vi "Edit Options.vi"(6 "Calling VI in":refnum<vi>, 8 "error in (no error)":errorcluster, 11 "Config":T1) -> (0 "error out":errorcluster, 2 "OK?":bool, 3 "Config out":T1)   [LabVIEW 2020, in "VI Properties Editor.lvlib"]
doc: "Displays a window to edit various options present in the tool."
uses:
  VI Properties Editor.lvlib
  CTLs/Config.ctl
  CTLs/Filter Info.ctl
  CTLs/Filter Column.ctl
  CTLs/Filter Type.ctl
panel:
  in  "Tab Control":enum32{"View", "Dialog", "Copyright"}(tab)
  in  "Show Conpane Ctls Only?":bool caption="Show connector pane controls only"
  in  "Format Bold Tags?":bool caption="Format bold text tags"
  in  "Abbreviate Names?":bool caption="Abbreviate names"
  in  "Show Top-Level Ctls Only?":bool caption="Show top-level controls only"
  in  "Confirm Save?":bool caption="Confirm Save action"
  in  "Confirm Save All?":bool caption="Confirm Save All action"
  in  "Confirm Revert?":bool caption="Confirm Revert action"
  in  "Confirm Revert All?":bool caption="Confirm Revert All action"
  in  "Confirm Exit?":bool caption="Confirm Exit with Unsaved Changes action"
  in  "Copyright delimiter":string
  in  "Copyright path":path
  in  "Cancel":bool
  in  "OK":bool
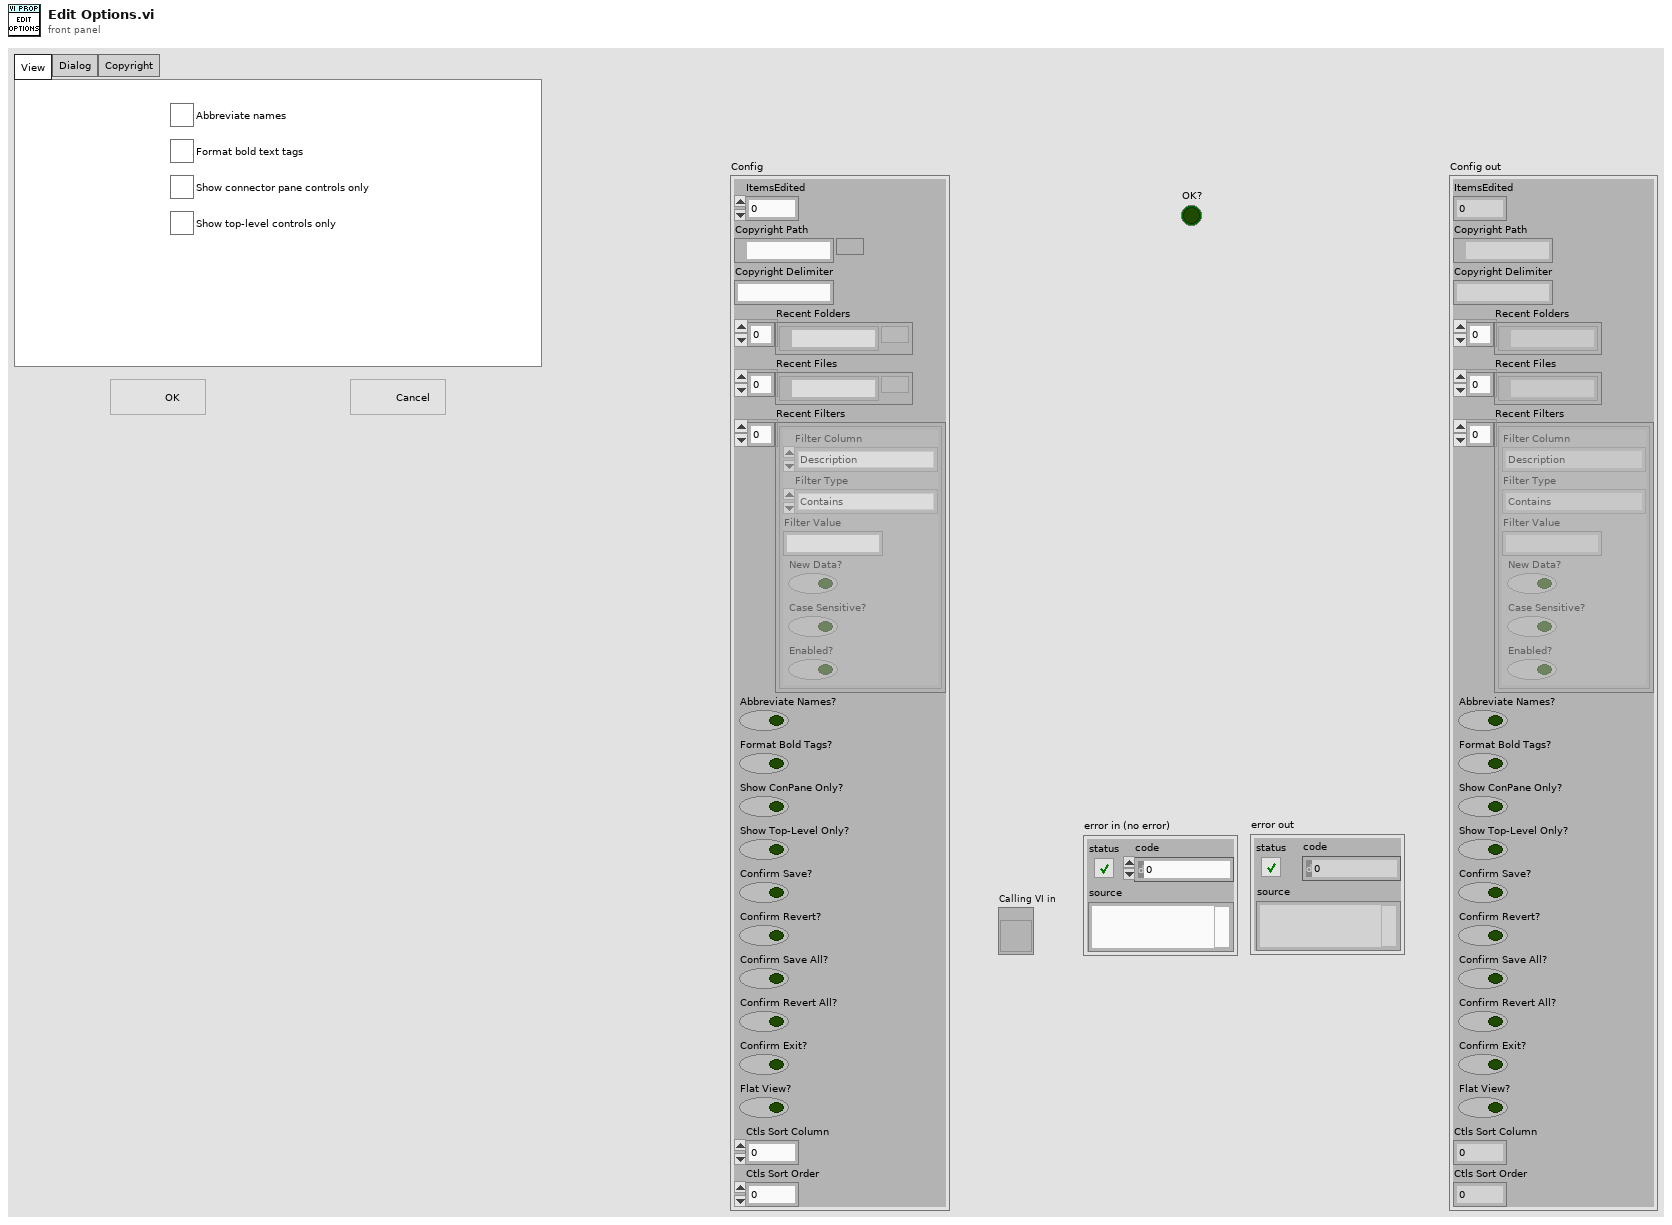
[diagram p1: front panel]
types:
  T1 = typedef "VI Properties Editor.lvlib/Config.ctl" = cluster{"ItemsEdited":u32, "Copyright Path":path, "Copyright Delimiter":string, "Recent Folders":path[], "Recent Files":path[], "Recent Filters":T2[], "Abbreviate Names?":bool, "Format Bold Tags?":bool, "Show ConPane Only?":bool, "Show Top-Level Only?":bool, "Confirm Save?":bool, "Confirm Revert?":bool, "Confirm Save All?":bool, "Confirm Revert All?":bool, "Confirm Exit?":bool, "Flat View?":bool, "Ctls Sort Column":i32, "Ctls Sort Order":i32}
  T2 = typedef "VI Properties Editor.lvlib/Filter Info.ctl" = cluster{"Filter Column":T3, "Filter Type":T4, "Filter Value":string, "New Data?":bool, "Case Sensitive?":bool, "Enabled?":bool}
  T3 = typedef "VI Properties Editor.lvlib/Filter Column.ctl" = enum16{"Name", "Path", "Type", "Window Title", "Description", "Help Path", "Help Tag", "Custom Title?", "Reentrancy", "Inlined?", "Help URL", "Help Type", "Allow Debugging?", "Auto Error Handling?", "Run When Opened?", "Suspend When Called?", "Priority", "Preferred Exec Sytem", "Control Label", "Control Caption", "Control Description", "Control Tip Strip"}
  T4 = typedef "VI Properties Editor.lvlib/Filter Type.ctl" = enum16{"Contains", "Equals", "Starts with", "Ends with", "Is empty", "Does not contain", "Does not equal", "Is not empty"}
  T5 = enum32{"Invalid", "Standard", "Closed", "Hidden", "Minimized", "Maximized"}
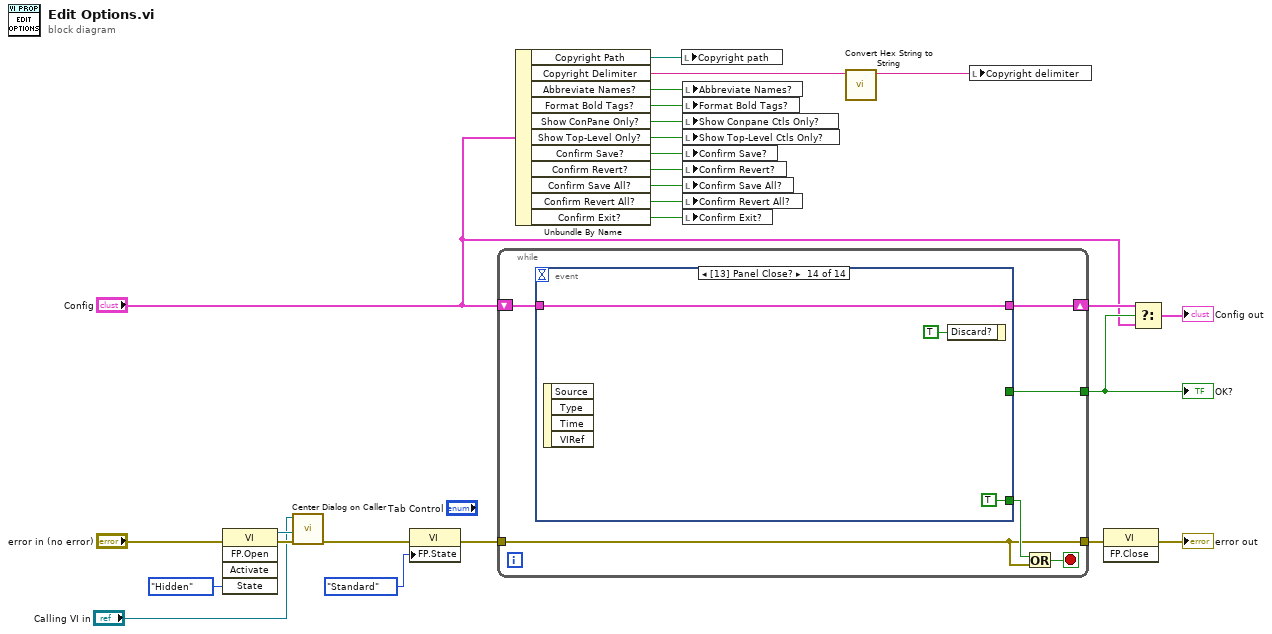
[diagram p0: block diagram]
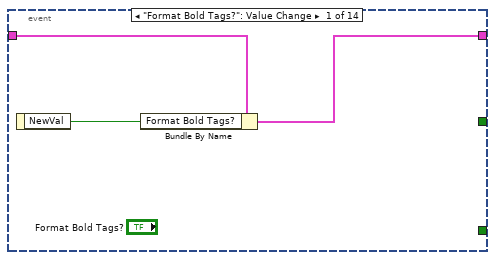
[diagram p2: hidden frame]
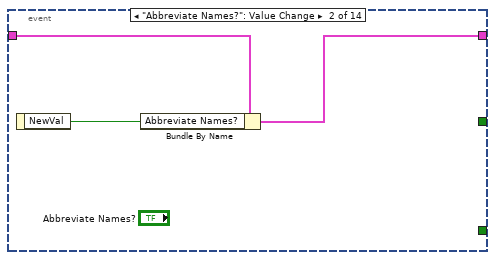
[diagram p3: hidden frame]
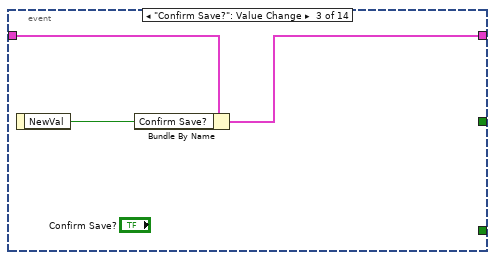
[diagram p4: hidden frame]
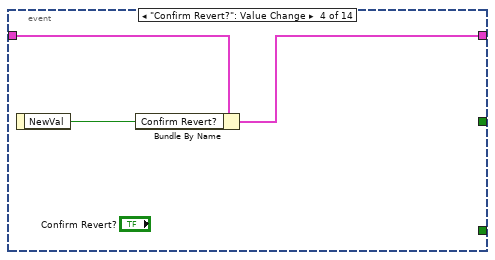
[diagram p5: hidden frame]
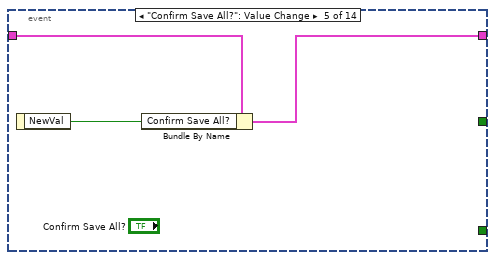
[diagram p6: hidden frame]
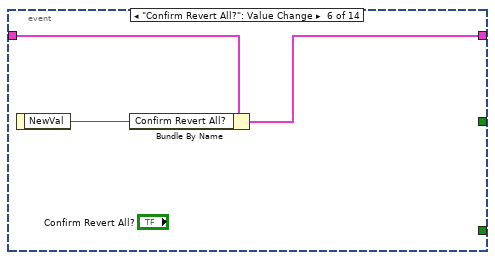
[diagram p7: hidden frame]
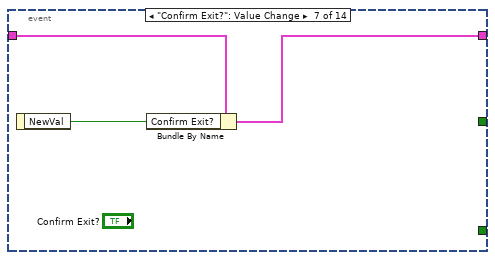
[diagram p8: hidden frame]
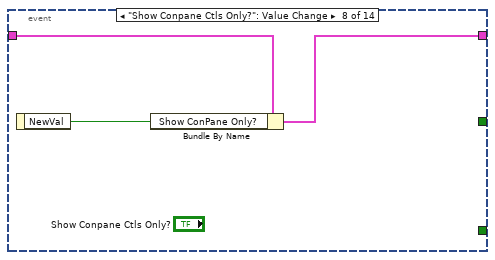
[diagram p9: hidden frame]
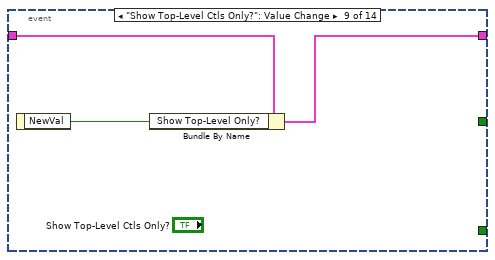
[diagram p10: hidden frame]
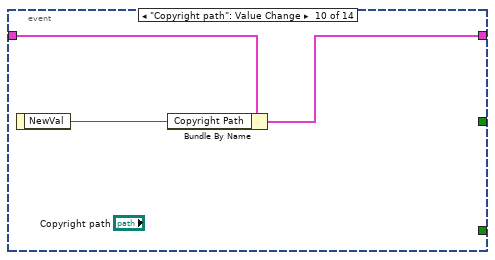
[diagram p11: hidden frame]
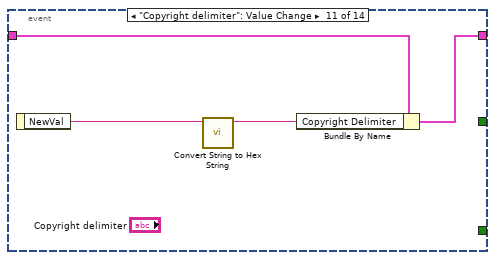
[diagram p12: hidden frame]
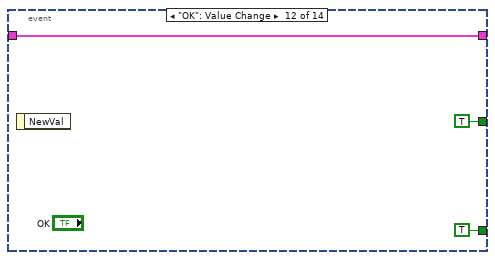
[diagram p13: hidden frame]
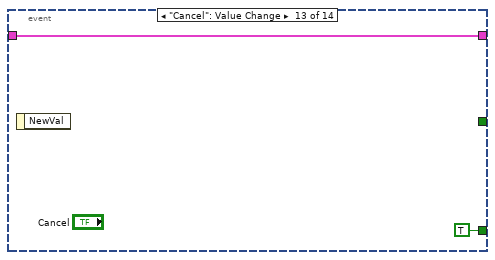
[diagram p14: hidden frame]
diagram:
  n1 = invoke class="VI" method="FP.Open"(error in="error in (no error)", "State"=T5."Hidden") -> (reference out=w11:refnum<vi>, error out=w12:errorcluster)  [unwired: 3 in, 3 out]
  n2 = call "Center Dialog on Caller.vi"("error in (no error)"=w12, "Dialog VI"=w11, "Calling VI in"="Calling VI in") -> ("error out"=w14:errorcluster)  [unwired: 7 in, 1 out]
  n3 = property class="VI"(error in=w14, "FP.State"=T5."Standard" ("Front Panel Window:State")) -> (error out=w7:errorcluster)  [unwired: 1 in, 1 out]
  n4 = while {
    shift-right: [w31] -> w19
    shift-left: "Config" -> [w32]
    tunnel: [w30] -> w18
    tunnel: w7 -> [w27]
    tunnel: [w27] -> w6
    stop <- w29 stop-if-true
    n5 = event shown="[13] Panel Close?" {
      selector: _ -> [_ _ _ _ _ _ _ _ _ _ _ _ _ _]
      dyn-events: _ -> [_ _ _ _ _ _ _ _ _ _ _ _ _ _]
      timeout: _ -> [_ _ _ _ _ _ _ _ _ _ _ _ _ _]
      tunnel: w32 -> [w35 w38 w41 w44 w47 w50 w53 w56 w59 w62 w66 w69 w71 w74]
      tunnel: [w33 w36 w39 w42 w45 w48 w51 w54 w57 w60 w65 w69 w71 w74] -> w31
      tunnel: [_ _ _ _ _ _ _ _ _ _ _ TRUE ("NewVal") _ _] -> w30
      tunnel: [_ _ _ _ _ _ _ _ _ _ _ TRUE ("NewVal") TRUE ("NewVal") TRUE ("NewVal")] -> w28
      event "Format Bold Tags?": Value Change {
        n6 = event-data() -> ("NewVal"=w34:bool)  [unwired: 1 in]
        n7 = Bundle By Name(cluster=w35, "Format Bold Tags?"=w34) -> (w33:T1)
      }
      event "Abbreviate Names?": Value Change {
        n8 = event-data() -> ("NewVal"=w37:bool)  [unwired: 1 in]
        n9 = Bundle By Name(cluster=w38, "Abbreviate Names?"=w37) -> (w36:T1)
      }
      event "Confirm Save?": Value Change {
        n10 = event-data() -> ("NewVal"=w40:bool)  [unwired: 1 in]
        n11 = Bundle By Name(cluster=w41, "Confirm Save?"=w40) -> (w39:T1)
      }
      event "Confirm Revert?": Value Change {
        n12 = event-data() -> ("NewVal"=w43:bool)  [unwired: 1 in]
        n13 = Bundle By Name(cluster=w44, "Confirm Revert?"=w43) -> (w42:T1)
      }
      event "Confirm Save All?": Value Change {
        n14 = event-data() -> ("NewVal"=w46:bool)  [unwired: 1 in]
        n15 = Bundle By Name(cluster=w47, "Confirm Save All?"=w46) -> (w45:T1)
      }
      event "Confirm Revert All?": Value Change {
        n16 = event-data() -> ("NewVal"=w49:bool)  [unwired: 1 in]
        n17 = Bundle By Name(cluster=w50, "Confirm Revert All?"=w49) -> (w48:T1)
      }
      event "Confirm Exit?": Value Change {
        n18 = event-data() -> ("NewVal"=w52:bool)  [unwired: 1 in]
        n19 = Bundle By Name(cluster=w53, "Confirm Exit?"=w52) -> (w51:T1)
      }
      event "Show Conpane Ctls Only?": Value Change {
        n20 = event-data() -> ("NewVal"=w55:bool)  [unwired: 1 in]
        n21 = Bundle By Name(cluster=w56, "Show ConPane Only?"=w55) -> (w54:T1)
      }
      event "Show Top-Level Ctls Only?": Value Change {
        n22 = event-data() -> ("NewVal"=w58:bool)  [unwired: 1 in]
        n23 = Bundle By Name(cluster=w59, "Show Top-Level Only?"=w58) -> (w57:T1)
      }
      event "Copyright path": Value Change {
        n24 = event-data() -> ("NewVal"=w61:path)  [unwired: 1 in]
        n25 = Bundle By Name(cluster=w62, "Copyright Path"=w61) -> (w60:T1)
      }
      event "Copyright delimiter": Value Change {
        n26 = event-data() -> ("NewVal"=w64:string)  [unwired: 1 in]
        n27 = call "Convert String to Hex String.vi"("String"=w64) -> ("Hex String"=w63:string)  [unwired: 10 in]
        n28 = Bundle By Name(cluster=w66, "Copyright Delimiter"=w63) -> (w65:T1)
      }
      event "OK": Value Change {
        n29 = event-data() -> ()  [unwired: 1 in, 1 out]
      }
      event "Cancel": Value Change {
        n30 = event-data() -> ()  [unwired: 1 in, 1 out]
      }
      event Panel Close? {
        n31 = event-data() -> ()  [unwired: 1 in, 4 out]
        n32 = event-data("Discard?"=TRUE) -> ()  [unwired: 1 in, 1 out]
      }
    }
    n33 = Or(x=w28, y=w27) -> (x .or. y?=w29:bool)
  }
  "OK?" <- w18
  n34 = Unbundle By Name("Config") -> ("Copyright Path"=w3:path, "Copyright Delimiter"=w2:string, "Abbreviate Names?"=w20:bool, "Format Bold Tags?"=w26:bool, "Show ConPane Only?"=w25:bool, "Show Top-Level Only?"=w4:bool, "Confirm Save?"=w24:bool, "Confirm Revert?"=w23:bool, "Confirm Save All?"=w22:bool, "Confirm Revert All?"=w21:bool, "Confirm Exit?"=w15:bool)
  n35 = local write "Copyright path"(w3) -> ()
  n36 = local write "Abbreviate Names?"(w20) -> ()
  n37 = local write "Format Bold Tags?"(w26) -> ()
  n38 = local write "Show Conpane Ctls Only?"(w25) -> ()
  n39 = local write "Show Top-Level Ctls Only?"(w4) -> ()
  n40 = local write "Confirm Save?"(w24) -> ()
  n41 = local write "Confirm Revert?"(w23) -> ()
  n42 = local write "Confirm Save All?"(w22) -> ()
  n43 = local write "Confirm Revert All?"(w21) -> ()
  n44 = local write "Confirm Exit?"(w15) -> ()
  n45 = call "Convert Hex String to String.vi"("Hex String"=w2) -> ("String"=w1:string)  [unwired: 10 in]
  n46 = local write "Copyright delimiter"(w1) -> ()
  n47 = invoke class="VI" method="FP.Close"(error in=w6) -> (error out=→"error out":errorcluster)  [unwired: 2 in, 2 out]
  n48 = Select(t=w19, s=w18, f="Config") -> (s? t:f=→"Config out":T1)
